vi "Build State String with Arguments++.vi"(5 "State":string, 7 "Arguments (\"\")":string, 9 "Target Module (\"\")":string, 12 "Type":T1) -> (6 "State with Arguments":string)   [LabVIEW 2014, in "JKI State Machine++.lvlib"]
doc: "Builds a state string that contains arguments for the JKI State Machine.\n\n<B>For Example:</B>\n\nFor local JKISM, <b>Target Module (\"\")</b> is empty.\n\n If State = A and no argument, then <b>State with Arguments</b> = A\n If State = A and Arguments = B then <b>State with Arguments</b> = A >> B\n\nFor sending message to other JKISM, suppose <b>Target Module (\"\")</b> is \"Target\"\n\n - For Sync-Call:\n\n If State = A and no argument, then <b>State with Arguments</b> = A -@target\n If State = A and Arguments = B then <b>State with Arguments</b> = A >> B -@target\n\n - For Async-Call:\n\n If State = A and no argument, then <b>State with Arguments</b> = A ->target\n If State = A and Arguments = B then <b>State with Arguments</b> = A >> B ->target\n\n<b>Inputs:</b>\n - <b>State</b>: The State or message string\n - <b>Arguments (\"\")</b>: The argument for <b>State</b>\n - <b>Target Module (\"\")</b>: The target JKISM module for the message to be sent to.\n - <b>Sync-Call(-@) T By Default/Async-Call(->) F</b>: For sync call, use \"TRUE\"; For Async call, use \"FALSE\"\n\n<b>Outputs:</b>\n - <b>State with Arguments</b>: String stands for state with arguments"
uses:
  JKI State Machine++.lvlib
  AdvanceAPI/JKISM++ Message Type.ctl
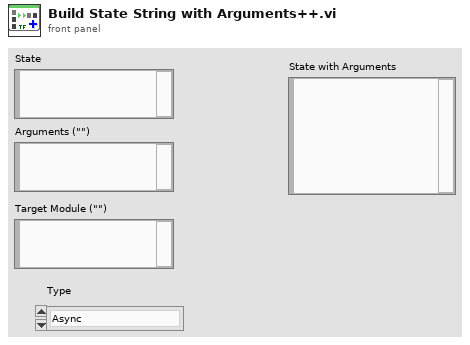
[diagram p1: front panel]
types:
  T1 = typedef "JKI State Machine++.lvlib/JKISM++ Message Type.ctl" = enum16{"Async", "Async without Reply", "Sync"}
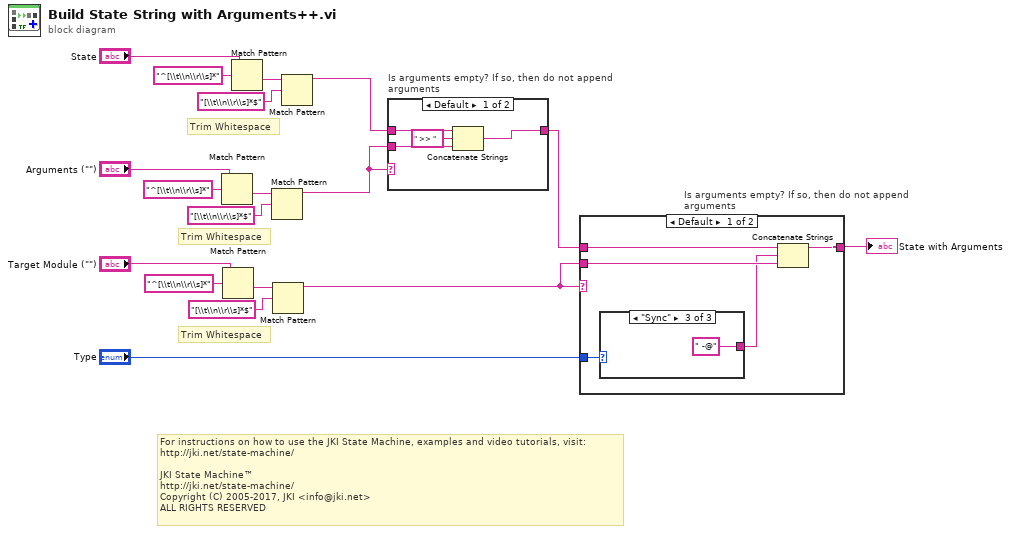
[diagram p0: block diagram]
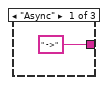
[diagram p2: hidden frame]
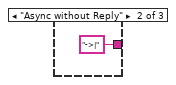
[diagram p3: hidden frame]
diagram:
  # "Trim Whitespace"
  # "Trim Whitespace"
  # "For instructions on how to use the JKI State Machine, examples and video tutorials, visit:\nhttp://jki.net/state-machine/\n\nJKI State Machine™\nhttp://jki.net/state-machine/\nCopyright (C) 2005-2017, JKI <info@jki.net>\nALL RIGHTS RESERVED"
  # "Trim Whitespace"
  n1 = Match Pattern(string="Arguments (\"\")", regular expression="^[\\t\\n\\r\\s]*") -> (after substring=w12:string)  [unwired: 1 in, 3 out]
  n2 = Match Pattern(string="Target Module (\"\")", regular expression="^[\\t\\n\\r\\s]*") -> (after substring=w7:string)  [unwired: 1 in, 3 out]
  n3 = Match Pattern(string="State", regular expression="^[\\t\\n\\r\\s]*") -> (after substring=w17:string)  [unwired: 1 in, 3 out]
  n4 = Match Pattern(string=w12, regular expression="[\\t\\n\\r\\s]*$") -> (before substring=w9:string)  [unwired: 1 in, 3 out]
  n5 = Match Pattern(string=w7, regular expression="[\\t\\n\\r\\s]*$") -> (before substring=w4:string)  [unwired: 1 in, 3 out]
  n6 = Match Pattern(string=w17, regular expression="[\\t\\n\\r\\s]*$") -> (before substring=w14:string)  [unwired: 1 in, 3 out]
  n7 = case "Is arguments empty? If so, then do not append arguments" shown="Default" w9 {
    tunnel: [w19 w23] -> w2
    tunnel: w14 -> [w22 w23]
    tunnel: w9 -> [w20 _]
    frame Default {
      n8 = Concatenate Strings(w22, " >> " ("string"), w20) -> (w19:string)
    }
    frame "" {
    }
  }
  n9 = case "Is arguments empty? If so, then do not append arguments" shown="Default" w4 {
    tunnel: [w26 w32] -> w3
    tunnel: w2 -> [w28 w32]
    tunnel: w4 -> [w27 _]
    tunnel: "Type" -> [w25 _]
    frame Default {
      n10 = case shown="\"Sync\"" w25 {
        tunnel: [" ->" ("string") "->|" ("string") " -@" ("string")] -> w24
        frame "Async" {
        }
        frame "Async without Reply" {
        }
        frame "Sync" {
        }
      }
      n11 = Concatenate Strings(w28, w24, w27) -> (w26:string)
    }
    frame "" {
    }
  }
  "State with Arguments" <- w3
